vi "InitSensors.vi"   [LabVIEW 2020]
doc: "This VI initializes independent sensing devices."
uses:
  refnumbers.vi
  <vilib>/Rock Robotics/WPI/ThirdParty/Phoenix-LabVIEW/Pigeon IMU/CTRE_PigeonIMU_Open_CAN.vi
  <vilib>/Rock Robotics/SystemInterfaces/i2clib/i2c_bus.ctl
types:
  T1 = typedef "i2c_bus.ctl" = enum16{"I2C On-Board", "I2C MXP", "Invalid"}
  T2 = typedef "CTRE_PigeonIMU_DeviceRef.ctl" = cluster{"DeviceStatus":errorcluster, "Device Number":u8, "Type":T3, "Device ID":u32, "Handle":u64, "UsageFrame":u32, "Library Path":path}
  T3 = typedef "CTRE_PigeonIMU_ConnectionType.ctl" = u32
  T4 = typedef "Color Sensor V3 DevRef.ctl" = cluster{"I2CDevRef":T5}
  T5 = typedef "WPI_I2CDevRef.ctl" = cluster{"DevStatus":errorcluster, "Device Address":u8, "Handle":i32, "I2C Bus":T1}
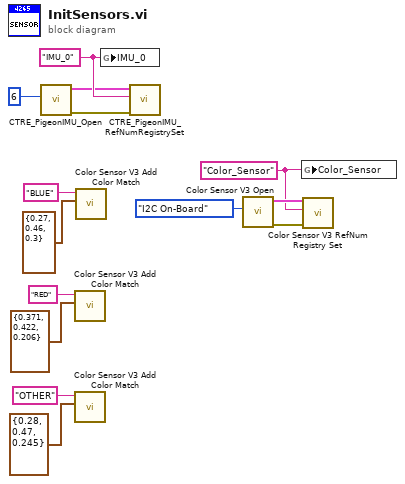
[diagram p0: block diagram]
diagram:
  w1 = "Color_Sensor" ("refnum name")
  w14 = "IMU_0" ("refnum name")
  n1 = call-poly <vilib>:"CTRE_PigeonIMU_Open.vi"("Device Number"=u8 6) -> ("error out"=w11:errorcluster, "PigeonIMUDevRef"=w12:T2)  [unwired: 9 in]
  n2 = call <vilib>:"Color Sensor V3 Add Color Match.vi"("Color"=cluster{"R":dbl, "G":dbl, "B":dbl} {"R"=0.371, "G"=0.422, "B"=0.206}, "Name"="RED") -> ()  [unwired: 10 in]
  n3 = call <vilib>:"Color Sensor V3 Add Color Match.vi"("Color"=cluster{"R":dbl, "G":dbl, "B":dbl} {"R"=0.28, "G"=0.47, "B"=0.245}, "Name"="OTHER") -> ()  [unwired: 10 in]
  n4 = call <vilib>:"Color Sensor V3 Add Color Match.vi"("Color"=cluster{"R":dbl, "G":dbl, "B":dbl} {"R"=0.27, "G"=0.46, "B"=0.3}, "Name"="BLUE") -> ()  [unwired: 10 in]
  n5 = global write "refnumbers.vi" "IMU_0"(w14) -> ()
  n6 = call <vilib>:"CTRE_PigeonIMU_RefNumRegistrySet.vi"("error in (no error)"=w11, "refnum name"=w14, "PigeonIMUDevRef"=w12) -> ()  [unwired: 7 in, 2 out]
  n7 = call <vilib>:"Color Sensor V3 Open.vi"("I2C Bus"=i2c_bus."I2C On-Board") -> ("error out"=w4:errorcluster, "ColorSensorDevRef"=w3:T4)  [unwired: 9 in]
  n8 = global write "refnumbers.vi" "Color_Sensor"(w1) -> ()
  n9 = call <vilib>:"Color Sensor V3 RefNum Registry Set.vi"("error in (no error)"=w4, "refnum name"=w1, "ColorSensorDevRef"=w3) -> ()  [unwired: 7 in, 2 out]
